vi "Teleop.vi"(10 "Match Info":T1={"Autonomous Elapsed Seconds"=0.0, "TeleOp Elapsed Seconds"=0.0, "Disabled Elapsed Seconds"=0.0, "Visited Autonomous"=FALSE, "Visited TeleOp"=FALSE, "Visited Disabled"=FALSE, "Autonomous Settings"={"Autonomous Style"=enum."Independent", "VI Refnum"=refnum}}, 11 "Call Context":T2) -> ()   [LabVIEW 2016]
doc: "This VI is called for each TeleOp packet received from the DS where the robot is not disabled. It is often used to read from the joysticks and update I/O or to update setpoints for timed control loops. It should complete and return within 20 milliseconds or it may miss DS packets."
uses:
  <vilib>/Rock Robotics/WPI/DriverStation/WPI_DriverStationDerivedRobotMode.ctl
  <vilib>/Rock Robotics/WPI/DriverStation/WPI_DriverStationMatch Info.ctl
  Robot Global Data.vi
  Global 4.vi
  <vilib>/Rock Robotics/WPI/Utilities/WPI_GetSetVariantRefNum.vi
  <vilib>/Rock Robotics/WPI/RobotDrive/WPI_RobotDriveMecanumDrive_Cartesian.vi
  <vilib>/Rock Robotics/Network Tables/NT Write Numeric Array.vi
  <vilib>/Rock Robotics/Network Tables/NT Write Boolean Array.vi
  <vilib>/Rock Robotics/Network Tables/NT Read Number.vi
  <vilib>/Rock Robotics/Network Tables/NT Read Boolean.vi
panel:
  out "Sample Slider 0":dbl(slide) scale=0.0..5.0
  out "Sample Boolean 1":bool
  out "Sample Boolean 0":bool
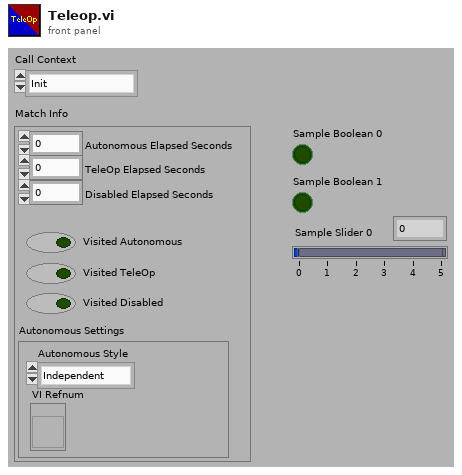
[diagram p1: front panel]
types:
  T1 = typedef "WPI_DriverStationMatch Info.ctl" = cluster{"Autonomous Elapsed Seconds":dbl, "TeleOp Elapsed Seconds":dbl, "Disabled Elapsed Seconds":dbl, "Visited Autonomous":bool, "Visited TeleOp":bool, "Visited Disabled":bool, "Autonomous Settings":cluster{"Autonomous Style":enum16{"Iterative", "Independent"}, "VI Refnum":refnum<vi>}}
  T2 = typedef "WPI_DriverStationDerivedRobotMode.ctl" = enum16{"Init", "Execute", "Stop"}
  T3 = typedef "WPI_RobotDriveDevRef.ctl" = cluster{"DevStatus":errorcluster, "Motors[]":T4[], "Square Inputs":bool, "Max Output":dbl}
  T4 = typedef "WPI_MotorControlDeviceRef.ctl" = cluster{"DeviceStatus":errorcluster, "Type":T5, "PWM":cluster{"PWM Channel":T6, "DeadBand":T7}, "CAN":cluster{"Device Number":u8, "SetOutput VI Ref":variant, "GetOutput VI Ref":variant, "Enable VI Ref":variant, "Disable VI Ref":variant, "Data":variant}, "Invert":bool}
  T5 = typedef "WPI_MotorControlType.ctl" = enum16{"PWM", "CAN"}
  T6 = typedef "FPGA_DIOPWMChannel.ctl" = enum8{"PWM 0", "PWM 1", "PWM 2", "PWM 3", "PWM 4", "PWM 5", "PWM 6", "PWM 7", "PWM 8", "PWM 9", "PWM MXP 0", "PWM MXP 1", "PWM MXP 2", "PWM MXP 3", "PWM MXP 4", "PWM MXP 5", "PWM MXP 6", "PWM MXP 7", "PWM MXP 8", "PWM MXP 9", "Invalid"}
  T7 = typedef "WPI_PWMDeadband.ctl" = cluster{"Name":string, "maxPositivePwm":i32, "minPositivePwm":i32, "centerPwm":i32, "maxNegativePwm":i32, "minNegativePwm":i32, "angularRange":u16}
  T8 = typedef "WPI_JoystickDevRef.ctl" = cluster{"Device":T9}
  T9 = typedef "WPI_JoystickDeviceEnum.ctl" = enum16{"USB 0", "USB 1", "USB 2", "USB 3", "USB 4", "USB 5"}
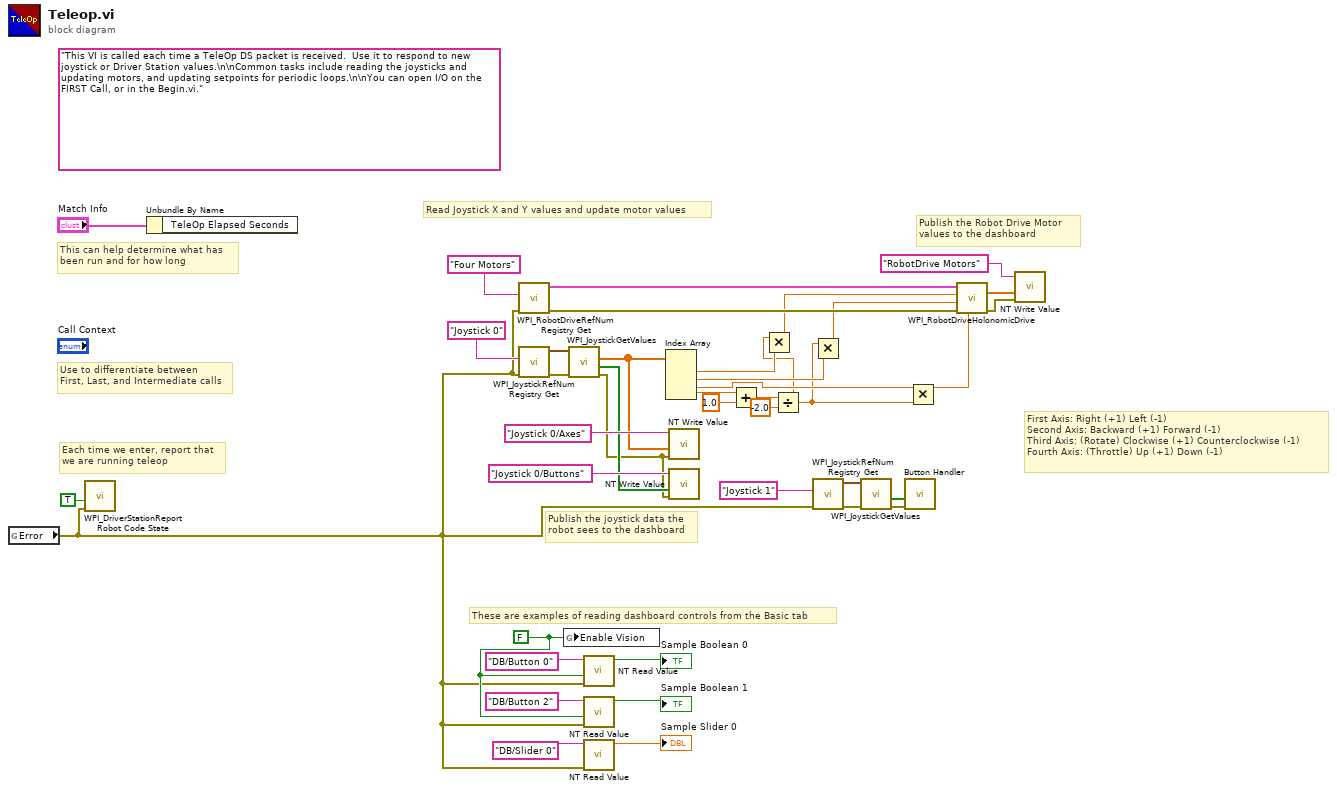
[diagram p0: block diagram]
diagram:
  w15 = FALSE
  (unwired) "This VI is called each time a TeleOp DS packet is received.  Use it to respond to new joystick or Driver Station values.\n\nCommon tasks include reading the joysticks and updating motors, and updating setpoints for periodic loops.\n\nYou can open I/O on the FIRST Call, or in the Begin.vi."
  # "First Axis: Right (+1) Left (-1)\nSecond Axis: Backward (+1) Forward (-1)\nThird Axis: (Rotate) Clockwise (+1) Counterclockwise (-1)\nFourth Axis: (Throttle) Up (+1) Down (-1)"
  # "These are examples of reading dashboard controls from the Basic tab"
  # "Publish the Robot Drive Motor\nvalues to the dashboard"
  # "Publish the joystick data the\nrobot sees to the dashboard"
  # "Each time we enter, report that\nwe are running teleop"
  # "Use to differentiate between\nFirst, Last, and Intermediate calls"
  # "This can help determine what has\nbeen run and for how long"
  # "Read Joystick X and Y values and update motor values"
  n1 = global read "Global 4.vi" "Error"() -> (w14:errorcluster)
  n2 = call <vilib>:"WPI_DriverStationReport Robot Code State.vi"("error in (no error)"=w14, "TeleOp"=TRUE ("Autonomous")) -> ()  [unwired: 9 in, 1 out]
  n3 = Unbundle By Name("Match Info") -> ()  [unwired: 1 out]
  n4 = call <vilib>:"WPI_RobotDriveRefNum Registry Get.vi"("error in (no error)"=w14, "refnum name"="Four Motors") -> ("error out"=w17:errorcluster, "RobotDriveDevRef"=w38:T3)  [unwired: 8 out]
  n5 = call <vilib>:"WPI_JoystickRefNum Registry Get.vi"("error in (no error)"=w14, "refnum name"="Joystick 0") -> ("error out"=w19:errorcluster, "JoystickDevRef"=w35:T8)  [unwired: 8 out]
  n6 = global write "Robot Global Data.vi" "Enable Vision"(w15) -> ()
  n7 = call <vilib>:"WPI_JoystickGetValues.vi"("error in (no error)"=w19, "JoystickDevRef"=w35) -> ("error out"=w18:errorcluster, "Buttons"=w26:bool[], "Axes"=w30:dbl[])  [unwired: 5 in, 2 out]
  n8 = call-poly <vilib>:"NT Read Value.vi"("error in"=w14, "Default Value"=w15, "Name"="DB/Button 0" ("refnum name")) -> ("Boolean"=→"Sample Boolean 0":bool)  [unwired: 7 in, 1 out]
  n9 = call-poly <vilib>:"NT Read Value.vi"("error in"=w14, "Default Value"=w15, "Name"="DB/Button 2" ("refnum name")) -> ("Boolean"=→"Sample Boolean 1":bool)  [unwired: 7 in, 1 out]
  n10 = call-poly <vilib>:"NT Read Value.vi"("error in"=w14, "Name"="DB/Slider 0" ("refnum name")) -> ("Numeric"=→"Sample Slider 0":dbl)  [unwired: 8 in, 1 out]
  n11 = Index Array(array=w30) -> (element #1=w37:dbl, element #2=w32:dbl, element #3=w33:dbl, element #4=w8:dbl)  [unwired: 4 in]
  n12 = call-poly <vilib>:"NT Write Value.vi"("error in"=w18, "Numeric Array"=w30, "Name"="Joystick 0/Axes") -> ()  [unwired: 8 in, 1 out]
  n13 = call-poly <vilib>:"NT Write Value.vi"("error in"=w18, "Boolean Array"=w26, "Name"="Joystick 0/Buttons") -> ()  [unwired: 8 in, 1 out]
  n14 = Add(x=w8, y=1.0) -> (x+y=w6:dbl)
  n15 = Divide(x=w6, y=-2.0) -> (x/y=w1:dbl)
  n16 = Multiply(x=w1, y=w37) -> (x*y=w4:dbl)
  n17 = Multiply(x=w1, y=w32) -> (x*y=w3:dbl)
  n18 = call <vilib>:"WPI_JoystickRefNum Registry Get.vi"("error in (no error)"=w14, "refnum name"="Joystick 1") -> ("error out"=w11:errorcluster, "JoystickDevRef"=w12:T8)  [unwired: 8 in]
  n19 = call <vilib>:"WPI_JoystickGetValues.vi"("error in (no error)"=w11, "JoystickDevRef"=w12) -> ("error out"=w9:errorcluster, "Buttons"=w10:bool[])  [unwired: 5 in, 3 out]
  n20 = call "Button Handler.vi"("error in (no error)"=w9, "Buttons"=w10) -> ()  [unwired: 9 in, 1 out]
  n21 = Multiply(x=w33, y=w1) -> (x*y=w2:dbl)
  n22 = call-poly <vilib>:"WPI_RobotDriveHolonomicDrive.vi"("Rotation"=w2, "error in (no error)"=w17, "Y"=w3, "X"=w4, "RobotDriveDevRef"=w38) -> ("error out"=w16:errorcluster, "Motor Values"=w28:dbl[])  [unwired: 4 in, 1 out]
  n23 = call-poly <vilib>:"NT Write Value.vi"("error in"=w16, "Numeric Array"=w28, "Name"="RobotDrive Motors") -> ()  [unwired: 8 in, 1 out]
